vi "Get Board Properties.vi"(8 "error in":errorcluster, 11 "custom device ref":T2 format="%.0x") -> (0 "error out":errorcluster, 2 "board properties out":T1 {"portConfig" items=["FDX_SINGLE", "FDX_REDUNDANT"]; "portSpeed" items=["FDX_100MBIT", "FDX_10MBIT", "FDX_AUTO_100MBIT", "FDX_AUTO_10MBIT", "FDX_AUTO_ERROR", "FDX_1000MBIT"]}, 3 "custom device ref out":T2 format="%.0x")   [LabVIEW 2020, in "AIM ARINC 664 Scripting.lvlib"]
uses:
  AIM ARINC 664 Scripting.lvlib
  <vilib>/NI VeriStand/Custom Device API/Custom Device Item Ref.ctl
  Import/_typedefs/board_setup.ctl
  Import/AIM ARINC 664 Import.lvlib
  <vilib>/NI VeriStand/Custom Device API/Custom Device API.lvlib
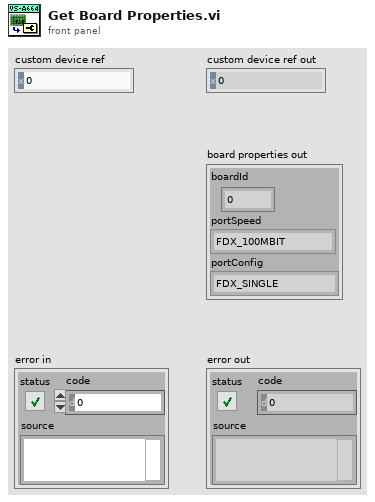
[diagram p1: front panel]
types:
  T1 = typedef "AIM ARINC 664 Import.lvlib/board_setup.ctl" = cluster{"boardId":u32, "portSpeed":u32, "portConfig":u32}
  T2 = typedef "Custom Device API.lvlib/Custom Device Item Ref.ctl" = u64
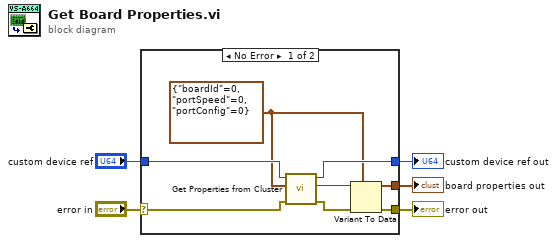
[diagram p0: block diagram]
diagram:
  n1 = case shown="No Error" "error in" {
    selector: "error in" -> [w6 w15]
    tunnel: "custom device ref" -> [w13 w14]
    tunnel: [w12 w14] -> w4
    tunnel: [w8 w15] -> w3
    tunnel: [w7 _] -> w2
    frame No Error {
      w11 = T1 {"boardId"=0, "portSpeed"=0, "portConfig"=0} ("boardSetup")
      n2 = call "Get Properties from Cluster.vi"("error in"=w6, "Variant Cluster"=w11, "custom device ref in"=w13) -> ("error out"=w9:errorcluster, "data"=w10:variant, "custom device ref out"=w12:T2)  [unwired: 5 in, 1 out]
      n3 = Variant To Data(error in=w9, type=w11, Variant=w10) -> (data=w7:T1, error out=w8:errorcluster)
    }
    frame Error {
    }
  }
  "custom device ref out" <- w4
  "error out" <- w3
  "board properties out" <- w2
